vi "Shift Register.vi"() -> ()   [LabVIEW 2021]
panel:
  out "String 2":string
  out "String":string
  out "Array":dbl[](array[numeric])
  in  "y":dbl
  out "Numeric 2":dbl
  out "Numeric":dbl
  out "Count 4":i32
  out "Count 3":i32
  out "Count 2":i32
  out "Count":i32
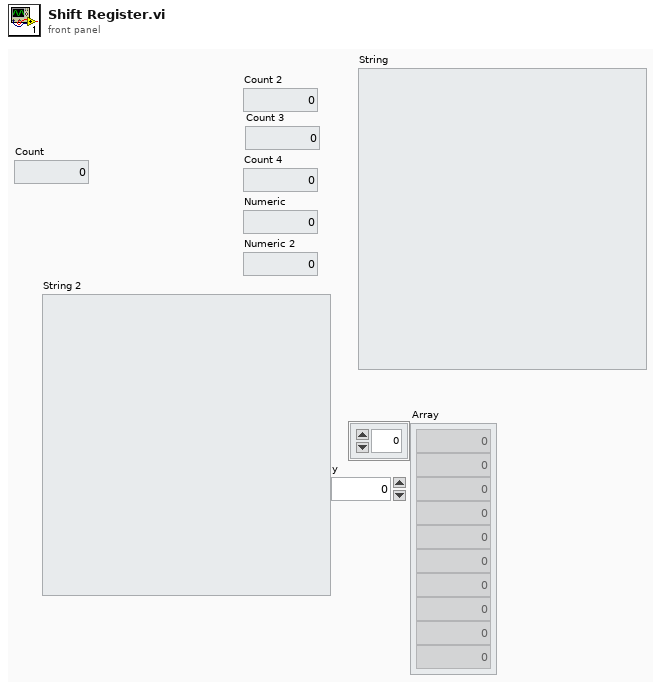
[diagram p1: front panel]
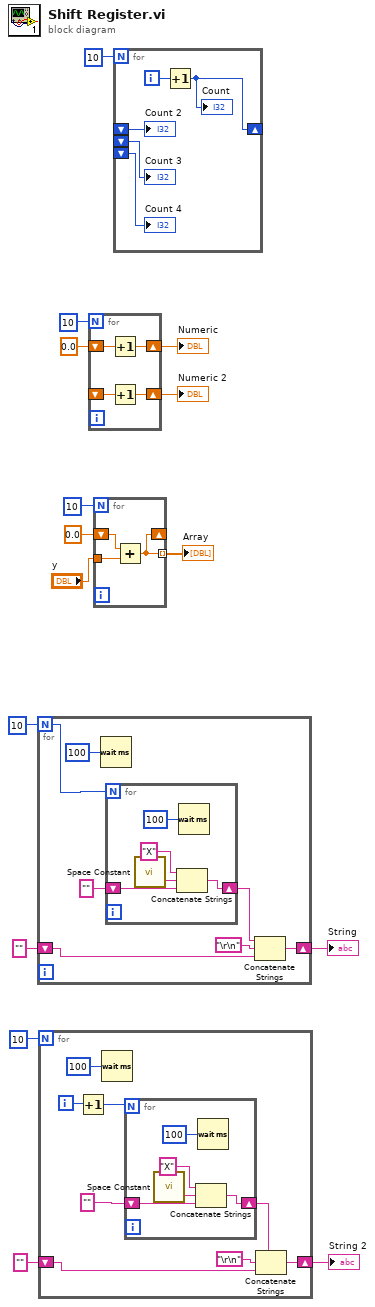
[diagram p0: block diagram]
diagram:
  n1 = for {
    N: 10 -> [w22]
    shift-right: [w17] -> w4
    shift-left: "" -> [w18]
    n2 = Wait (ms)(milliseconds to wait=u32 100) -> ()  [unwired: 1 out]
    n3 = for {
      N: w22 -> [_]
      shift-right: [w25] -> w20
      shift-left: "" -> [w24]
      n4 = call <vilib>:"Space Constant.vi"() -> ("String"=w26:string)
      n5 = Concatenate Strings("X", w26, w24) -> (w25:string)
      n6 = Wait (ms)(milliseconds to wait=u32 100) -> ()  [unwired: 1 out]
    }
    n7 = Concatenate Strings(w20, "\r\n", w18) -> (w17:string)
  }
  "String" <- w4
  n8 = for {
    N: 10 -> [_]
    shift-right: [w31] -> w1
    shift-left: "" -> [w32]
    i -> [w29]
    n9 = Increment(x=w29) -> (x+1=w28:i32)
    n10 = Wait (ms)(milliseconds to wait=u32 100) -> ()  [unwired: 1 out]
    n11 = for {
      N: w28 -> [_]
      shift-right: [w38] -> w34
      shift-left: "" -> [w37]
      n12 = call <vilib>:"Space Constant.vi"() -> ("String"=w39:string)
      n13 = Concatenate Strings("X", w39, w37) -> (w38:string)
      n14 = Wait (ms)(milliseconds to wait=u32 100) -> ()  [unwired: 1 out]
    }
    n15 = Concatenate Strings(w34, "\r\n", w32) -> (w31:string)
  }
  "String 2" <- w1
  n16 = for {
    N: 10 -> [_]
    shift-right: [w43] -> w13
    shift-left: 0.0 -> [w44]
    shift-right: [w41] -> w12
    shift-left: _ -> [w42]
    n17 = Increment(x=w44) -> (x+1=w43:dbl)
    n18 = Increment(x=w42) -> (x+1=w41:dbl)
  }
  "Numeric" <- w13
  "Numeric 2" <- w12
  n19 = for {
    N: 10 -> [_]
    shift-right: [w45] -> _
    shift-left: 0.0 -> [w47]
    tunnel: "y" -> [w46]
    tunnel: [w45] -> w7 mode=indexing
    n20 = Add(x=w47, y=w46) -> (x+y=w45:dbl)
  }
  "Array" <- w7
  n21 = for {
    N: 10 -> [_]
    shift-right: [w50] -> _
    shift-left: _ -> [w51]
    shift-left: _ -> [w49]
    shift-left: _ -> [w48]
    i -> [w52]
    n22 = Increment(x=w52) -> (x+1=w50:i32)
    "Count" <- w50
    "Count 2" <- w51
    "Count 3" <- w49
    "Count 4" <- w48
  }
